vi "Offline-Analysis.vi"() -> ()   [LabVIEW 2024]
uses:
  <vilib>/Utility/TDMS File Viewer/NI_TDMS File Viewer.lvlib
panel:
  out "Select File Path Analysis":path caption="Select File Path"
  # "Instructions:\n1.Run This vi\n2.TDMS file selection dialog shown to the user\n3.TDMS File Viewer then launches after file selection and displays the TDMS file content\n4.First showing a ‘File Loading…’ message and then displaying the selected file’s contents.\n5.By default, the viewer shows 10,000 samples. \n6.The user may also select the ‘All’ checkbox to load the complete dataset.\n7.A start index option allows the user to choose the starting row of samples. \n8.The viewer displays both the full data and any selected channels in graphical form as well as in tabular (array) form.\n9.The user can select multiple channels by holding the Ctrl key and clicking with the mouse."
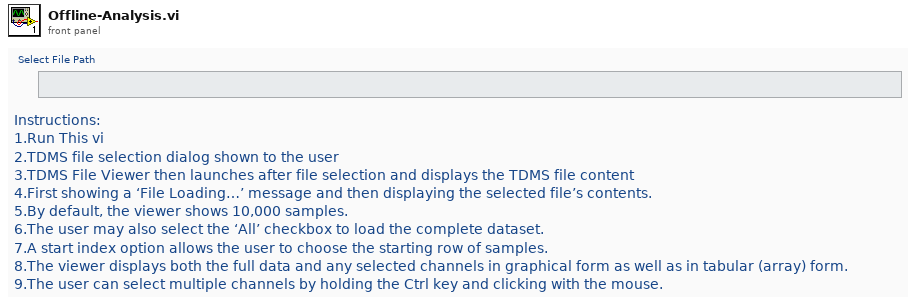
[diagram p1: front panel]
types:
  T1 = enum16{"open", "open or create", "create or replace", "create", "open (read-only)"}
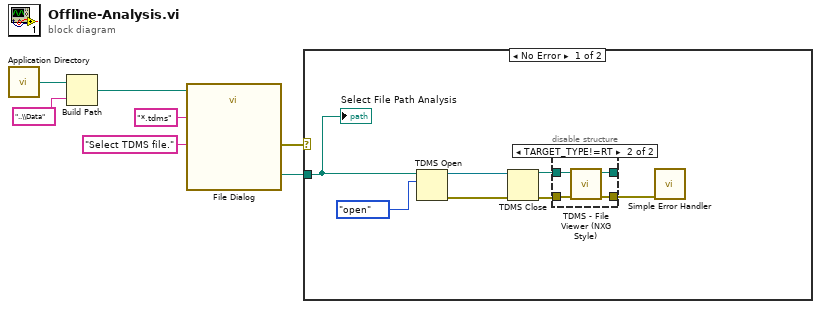
[diagram p0: block diagram]
diagram:
  n1 = call <vilib>:"Application Directory.vi"() -> ("Application Directory"=w7:path)
  n2 = Build Path(base path=w7, name or relative path="..\\Data") -> (appended path=w5:path)
  n3 = call "File Dialog"("start path"=w5, "prompt"="Select TDMS file.", "pattern (all files)"="*.tdms") -> ("selected path"=w2:path, "error out"=w1:errorcluster)  [unwired: 9 in, 2 out]
  n4 = case shown="No Error" w1 {
    tunnel: w2 -> [w8 _]
    frame No Error {
      n5 = TDMS Open(10:T1."open" ("operation"), 11:w8) -> (0:w10:errorcluster, 3:w9:refnum<k34>)  [unwired: 5 in]
      n6 = TDMS Close(8:w10, 11:w9) -> (0:w12:errorcluster, 3:w13:path)
      n7 = disable-structure shown="TARGET_TYPE!=RT" {
        disable-tunnel: w12 -> [w16 w20]
        disable-tunnel: w13 -> [w15 w19]
        disable-tunnel: [w16 w18] -> w11
        disable-tunnel: [w15 w17] -> _
        frame condition #0 {
        }
        frame condition #1 (active) {
          n8 = call <vilib>:"TDMS - File Viewer (NXG Style).vi"("error in"=w20, "file in"=w19) -> ("error out"=w18:errorcluster, "file out"=w17:path)  [unwired: 8 in]
        }
      }
      n9 = call <vilib>:"Simple Error Handler.vi"("error in (no error)"=w11) -> ()  [unwired: 4 in, 5 out]
      "Select File Path Analysis" <- w8
    }
    frame Error {
    }
  }
